vi "断电保存全局.vi"() -> ()   [LabVIEW 2016, in "数据传输系统.lvlib"]
panel:
  in  "数据重发时间戳":string="1994/10/09 09:20:28"
  out "数据重发":bool
  in  "数据组合发送":bool
  in  "日志、参数发送":bool
  in  "2011发送":bool
  in  "判断数据反馈":bool
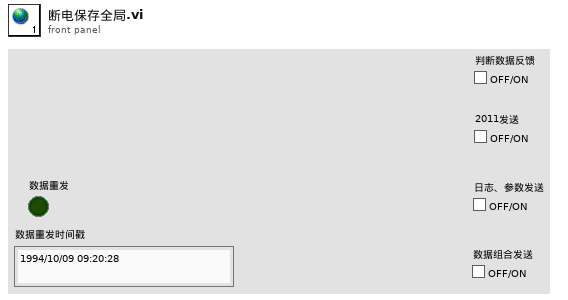
[diagram p1: front panel]
diagram:
